vi "Find Object Item Offsets by Names.vi"(7 "JSON Object":string, 9 "Offset":i32, 10 "Item Names <JSON>":string[](array[string])) -> (1 "Items":T1(array[cluster]), 3 "State":T2)   [LabVIEW 2013, in "JSON2.lvlib"]
uses:
  JSON2.lvlib
  JSON Value Search.ctl
  Advance past Number.vi
  Advance past Array.vi
  Advance past Object.vi
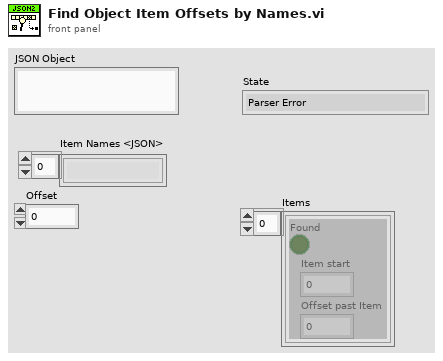
[diagram p1: front panel]
types:
  T1 = cluster{"Found":bool, "Item start":i32, "Offset past Item":i32}[]
  T2 = typedef "JSON2.lvlib/JSON Value Search.ctl" = enum16{"Parser Error", "In Object", "In Array", "String", "Number", "Leading Whitespace", "Object end", "Array end", "Value end", "Undefined"}
  T3 = cluster{"Found":bool, "Item start":i32, "Offset past Item":i32}
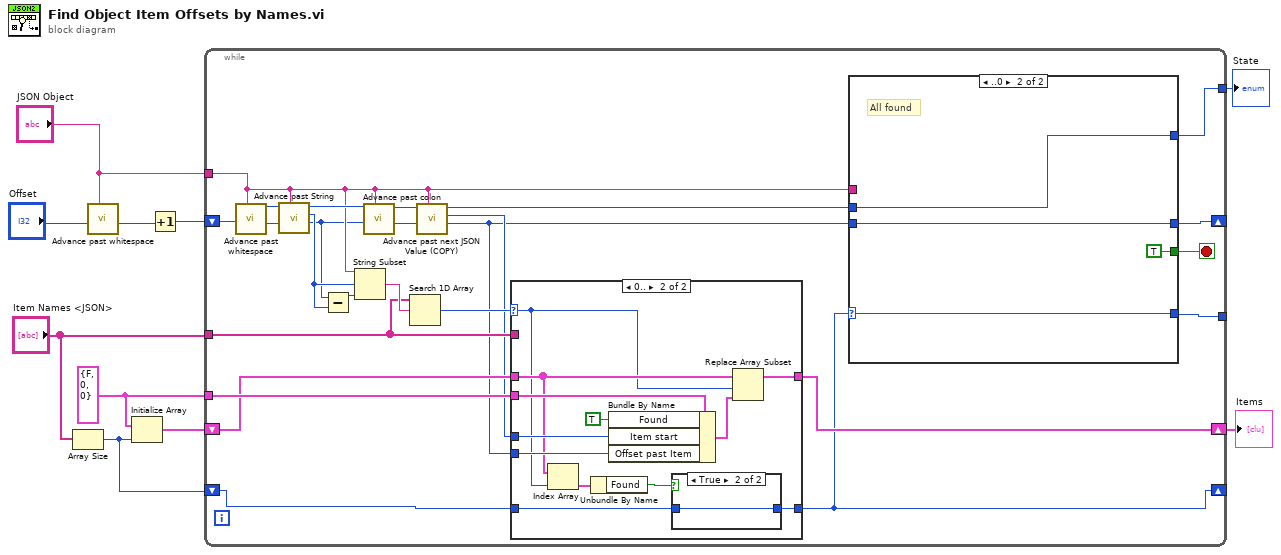
[diagram p0: block diagram]
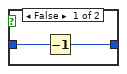
[diagram p3: hidden frame]
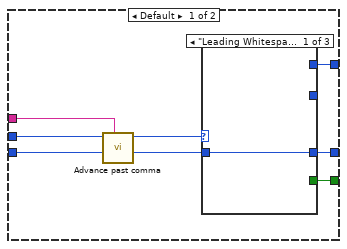
[diagram p4: hidden frame]
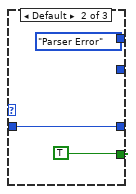
[diagram p5: hidden frame]
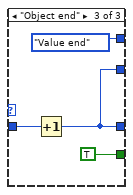
[diagram p6: hidden frame]
diagram:
  w3 = T3 {"Found"=FALSE, "Item start"=0, "Offset past Item"=0}
  n1 = Array Size(array="Item Names <JSON>") -> (size(s)=w2:i32)
  n2 = call "Advance past whitespace.vi"("JSON"="JSON Object", "Offset"="Offset") -> ("Offset past match"=w8:i32)  [unwired: 7 in, 2 out]
  n3 = Initialize Array(w3, w2) -> (w4:T1)
  n4 = Increment(x=w8) -> (x+1=w9:i32)
  n5 = while {
    shift-right: [w34] -> _
    shift-left: w9 -> [w31]
    tunnel: "JSON Object" -> [w25]
    tunnel: [w32] -> w10
    tunnel: "Item Names <JSON>" -> [w17]
    tunnel: [w23] -> _
    tunnel: w3 -> [w21]
    shift-right: [w15] -> w1
    shift-left: w4 -> [w16]
    shift-right: [w13] -> _
    shift-left: w2 -> [w14]
    stop <- w33 stop-if-true
    n6 = call "Advance past whitespace.vi"("JSON"=w25, "Offset"=w31) -> ("Offset past match"=w30:i32, "State"=w29:T2)  [unwired: 7 in, 1 out]
    n7 = call "Advance past String.vi"("JSON"=w25, "Offset"=w30, "State in"=w29) -> ("Offset past match"=w19:i32, "Value start out"=w20:i32, "State"=w35:T2)  [unwired: 6 in]
    n8 = Subtract(x=w19, y=w20) -> (x-y=w24:i32)
    n9 = String Subset(string=w25, offset (0)=w20, length (rest)=w24) -> (substring=w22:string)
    n10 = call "Advance past colon.vi"("JSON"=w25, "Offset"=w19, "State"=w35) -> ("index"=w26:i32, "State"=w27:T2)  [unwired: 7 in]
    n11 = Search 1D Array(1D array=w17, element=w22) -> (index of element=w18:i32)  [unwired: 1 in]
    n12 = call "Advance past next JSON Value (COPY).vi"("JSON"=w25, "Offset"=w26, "State"=w27) -> ("index"=w11:i32, "Value start"=w12:i32, "State"=w28:T2)  [unwired: 6 in]
    n13 = case shown="0.." w18 {
      selector: w18 -> [_ w43]
      tunnel: w21 -> [_ w49]
      tunnel: w12 -> [_ w47]
      tunnel: w11 -> [_ w46]
      tunnel: w17 -> [_ _]
      tunnel: w16 -> [w37 w44]
      tunnel: [w37 w42] -> w15
      tunnel: w14 -> [w36 w39]
      tunnel: [w36 w38] -> w13
      frame Default {
      }
      frame 0.. {
        n14 = Index Array(array=w44, index=w43) -> (element=w41:T3)
        n15 = Unbundle By Name(w41) -> ("Found"=w40:bool)
        n16 = Bundle By Name(cluster=w49, "Found"=TRUE, "Item start"=w47, "Offset past Item"=w46) -> (w45:T3)
        n17 = case shown="True" w40 {
          tunnel: w39 -> [w51 w52]
          tunnel: [w50 w52] -> w38
          frame False {
            n18 = Decrement(x=w51) -> (x-1=w50:i32)
          }
          frame True {
          }
        }
        n19 = Replace Array Subset(array=w44, new element=w45, index=w43) -> (w42:T1)
      }
    }
    n20 = case shown="..0" w13 {
      selector: w13 -> [_ w69]
      tunnel: [w59 w71] -> w34
      tunnel: [w58 TRUE] -> w33
      tunnel: [w57 w72] -> w32
      tunnel: w28 -> [w55 w72]
      tunnel: w11 -> [w54 w71]
      tunnel: w25 -> [w56 _]
      tunnel: [_ w69] -> w23
      frame Default {
        n21 = call "Advance past comma.vi"("JSON"=w56, "Offset"=w54, "State in"=w55) -> ("Offset past match"=w53:i32, "State"=w60:T2)  [unwired: 7 in]
        n22 = case shown="\"Leading Whitespace\"" w60 {
          tunnel: [_ TRUE TRUE] -> w58
          tunnel: [_ JSON_Value_Search."Parser Error" JSON_Value_Search."Value end"] -> w57
          tunnel: w53 -> [w61 w62 w66]
          tunnel: [w61 w62 w65] -> w59
          tunnel: [_ _ w65] -> _
          frame "Leading Whitespace" {
          }
          frame Default {
          }
          frame "Object end" {
            n23 = Increment(x=w66) -> (x+1=w65:i32)
          }
        }
      }
      frame ..0 {
        # "All found"
      }
    }
  }
  "State" <- w10
  "Items" <- w1
